vi "Test 3 Skipped Method.vi"(8 "error in (no error)":errorcluster, 11 "Test Test Case in":refnum<class "Skip and Pass Test Case.lvclass">) -> (0 "error out":errorcluster, 3 "Test Test Case out":refnum<class "Skip and Pass Test Case.lvclass">)   [LabVIEW 2020, in "Skip and Pass Test Case.lvclass"]
uses:
  Skip and Pass Test Case.lvclass
  Skip and Pass Test Case.lvclass/Skip and Pass Test Case.ctl
  source/Framework/Test Case/LUnit Test Case.lvclass
  C:/Git/astemes-lunit/source/Framework/Test Case/LUnit Test Case.lvclass
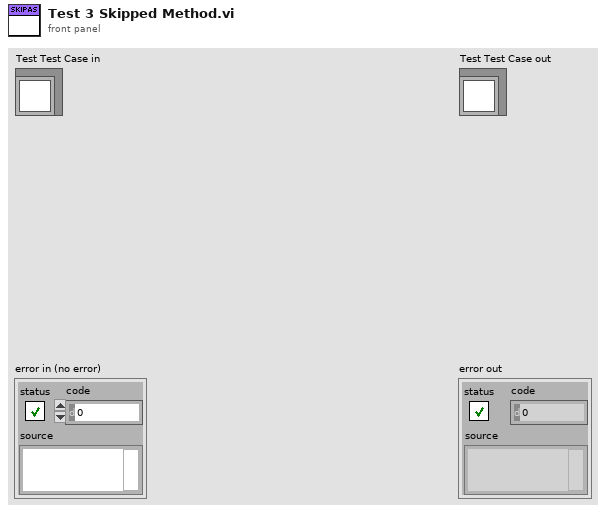
[diagram p1: front panel]
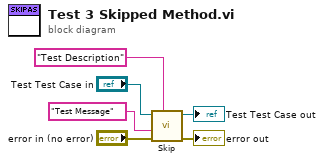
[diagram p0: block diagram]
diagram:
  n1 = call "Skip.vi"("Description"="Test Description", "error in (no error)"="error in (no error)", "Message"="Test Message", "LUnit Test Case In"="Test Test Case in") -> ("error out"=→"error out":errorcluster, "LUnit Test Case Out"=→"Test Test Case out":refnum<class "Skip and Pass Test Case.lvclass">)  [unwired: 6 in]
